vi "UHR-Fleezers Control (fpga) - 10.3 Troy.vi"() -> ()   [LabVIEW 2013]
doc: "UHR-Fleezers Instrument Control Code (fpga)"
uses:
  <vilib>/Platform/TimedLoop/XDataNode/timing_clust.ctl
  <vilib>/Platform/TimedLoop/XDataNode/nitl_modes.ctl
  <vilib>/Platform/TimedLoop/XDataNode/wakeup.ctl
  <vilib>/rvi/eio/common/nirviEmuTemplateMethod_errors.vi
  <vilib>/rvi/Emulation/niFpgaSctlEmulationGetInTimedLoop.vi
  <vilib>/rvi/Emulation/niFpgaEmulationReportErrorSimple.vi
  <vilib>/rvi/Emulation/niFpgaGetClockAttributes.vi
  <vilib>/rvi/Emulation/niFpgaCriticalErrorInLSC.vi
  <vilib>/rvi/Emulation/niFpgaProcessEmulError.vi
  <vilib>/rvi/interface/RandomDataEmulation/nirviRandomDataFPGAFIFO.vi
  <vilib>/rvi/interface/RandomDataEmulation/niFpgaRandomDataHandleErrors.vi
  <vilib>/Platform/TimedLoop/XDataNode/XDataNode.xnode
  <vilib>/eio/EIOMethodNode/EIOMethodNode.xnode
  <vilib>/eio/EIONode/EIONode.xnode
  <vilib>/rvi/DataTransferAndStorage/Container/XNode/niFpgaContainer.xnode
  <vilib>/rvi/interface/RandomDataEmulation/nirviRandomDataFpgaReadWriteTemplate.vi
  <vilib>/addons/control/pid/fpga.llb/XNode/niFpgaPID.xnode
  <vilib>/Platform/TimedLoop/XDataNode/XDNodeRunTimeDep.lvlib
panel:
  out "Trap Pos FB Int-Norm Signal":fxp<+/-,16,1> format="%.16g"
  out "Trap Pos FB Int Signal":fxp<+/-,24,9> format="%.18g"
  in  "Tab Control":T1(tab)
  in  "AI1 X Scale":u16
  in  "Trap Pos FB Monitor T1 or T2":bool
  in  "Trap Pos FB Negate Action":bool
  in  "Trap Pos. FB SP":fxp<+/-,16,1>
  in  "Trap Pos. FB Reset":bool
  in  "Trap Pos to FIFO":bool
  in  "AI1 Sets to FIFO":T2={"Set 1"=TRUE, "Set 2"=TRUE, "Set 3"=FALSE}
  in  "N of AI1 Int Acq Sets":i16=2 min=1 max=3 step=1
  out "AI Late Counter":u16
  in  "ai count":u32=400
  out "AI late?":bool
  in  "+ phase":bool
  in  "Phase count adjustment":i16
  out "Relative phase":i16
  in  "AI to FIFO":bool
  out "BD1 Frequency Out 1":u64
  out "BD1 Frequency Out 2":u64
  in  "Force feedback":bool
  out "AI1 X Set 1":fxp<+/-,16,1>
  in  "Trap Pos. FB Gains":T3={"proportional gain (Kc)"=0.0, "integral gain (Kc*Ts/Ti)"=10.0, "derivative gain (Kc*Td/Ts)"=0.0} {"proportional gain (Kc)" format="%.11g"; "integral gain (Kc*Ts/Ti)" format="%.11g"; "derivative gain (Kc*Td/Ts)" format="%.11g"}
  in  "Trap Pos. FB Range":T4={"output high"=0.999969482421875, "output low"=-1.0}
  in  "Trap Pos. FB Mult Factor":i64=2
  in  "Trap Pos. FB Offset Factor":i64
  out "AI1 X Set 2":fxp<+/-,16,1>
  out "Trap Pos FB Action":i64
  out "Trap Pos FIFO Timeout":u16
  out "Trap AI FIFO Timeout":u16
  in  "Trap FIFO Set Timeout":i32
  in  "Trap Pos FB Int Count":u16=100
  in  "Tab Control 2":T5(tab)
  in  "Swap F1 and F2":bool
  in  "Freq or Amp switch first":bool=TRUE
  in  "Cont. Scan":bool
  in  "Abort scan":bool
  in  "Cycles per step":u64
  in  "Scan BD":bool
  in  "Number of scans":u16
  in  "Scan steps":u64
  in  "Scan freq.  increment":i64
  out "Scanning":bool
  in  "Start scan":bool
  in  "OSK Bd 1":bool
  in  "Reset Bd 1":bool
  in  "RD":bool
  in  "PMODE":bool
  in  "OSK Bd 2":bool
  in  "Reset Bd 2":bool
  in  "Direct RF Box \nCommunication":bool
  in  "Data BD 2":u8 format="%08b"
  in  "Data BD 1":u8 format="%08b"
  in  "Address":u8 format="%02x"
  in  "Update Data":bool
  in  "FPGA Controls\n RF Box":bool
  in  "Number Interlace Cycles":u8=2 min=1 max=3
  in  "Interlace Off Parameters":u8=1 min=1 max=3
  in  "Interlace ON/OFF":bool
  out "DIO Relative phase":i16
  in  "Phase count adjustment (DIO)":i16
  in  "+ phase (DIO)":bool
  out "DIO Late Counter":u16
  out "DIO Late?":bool
  in  "DIO count 1 (ticks)":u32=400
  in  "DIO count 2 (ticks)":u32=400
  in  "DIO count 3 (ticks)":u32=400
  out "AI2 Y Sum Set 2":i16
  out "AI2 Y Sum Set 1":i16
  in  "FB Gains Set 1":T6={"proportional gain (Kc)"=10, "integral gain (Kc*Ts/Ti)"=5, "derivative gain (Kc*Td/Ts)"=0}
  in  "FB Setpoint Set 1":i16 min=0 step=1
  in  "FB Reset Set 1":bool
  in  "FB On/Off Set 1":bool
  in  "FB Reset Set 2":bool
  in  "FB On/Off Set 2":bool
  in  "FB Setpoint Set 2":i16 min=0 step=1
  in  "FB Gains Set 2":T6={"proportional gain (Kc)"=10, "integral gain (Kc*Ts/Ti)"=5, "derivative gain (Kc*Td/Ts)"=0}
  in  "FB output range 2":cluster{"output high":i16, "output low":i16}={"output high"=3000, "output low"=0}
  in  "FB output range 1":cluster{"output high":i16, "output low":i16}={"output high"=3000, "output low"=0}
  out "Scan I":u64
  in  "Amp switch delay":u16=5
  in  "Freq switch delay":u16
  in  "BD 2 Amplitude 1":u16
  in  "BD 1 Amplitude 1":u16
  in  "BD 2 Frequency 1":u64
  in  "BD 1 Frequency 1":u64
  in  "BD 2 Amplitude 2":u16
  in  "BD 1 Amplitude 2":u16
  in  "BD 2 Frequency 2":u64
  in  "BD 1 Frequency 2":u64
  in  "BD 2 Amplitude 3":u16
  in  "BD 1 Amplitude 3":u16
  in  "BD 2 Frequency 3":u64
  in  "BD 1 Frequency 3":u64
  out "Numeric":i32
  out "AO2 2":i16
  out "AO1 2":i16
  in  "1D or 2D Scan?":bool
  in  "Abort scan (MCL)":bool
  in  "MCL Scan Axis":bool
  in  "Cont. Scan (MCL)":bool
  out "Scan I (MCL)":u64
  in  "Number of scans (MCL)":u16
  out "Scanning MCL":bool
  in  "Scan steps (MCL)":u64
  in  "Cycles per step (MCL)":u64
  in  "Scan freq.  increment (MCL)":i16
  in  "Start scan (MCL)":bool
  in  "AO2":i16
  in  "AO1":i16
  out "MCL Late Counter":u16
  out "MCL Late?":bool
  in  "MCL count":u32=800
  out "MCL Relative Phase":i16
  in  "Phase count adjustment (MCL)":i16
  in  "+ phase (MCL)":bool
  in  "APD Gate Operating Mode":u8 max=2 step=1
  in  "Invert APD Gate":bool
  in  "APD Gate OFF Count":u32=100
  in  "APD Gate ON Count":u32=300
  out "APD 1 Gate Late Counter":u16
  out "APD 1 Gate Late?":bool
  out "APD 1 Gate Relative Phase":i16
  in  "Phase count adjustment (APD 1 Gate)":i16
  in  "+ phase (APD 1 Gate)":bool
  out "APD 2 Counts 0":u32
  out "APD 2 Counts 1":u32
  out "APD 1 Counts 0":u32
  out "APD 1 Counts 1":u32
  out "APD1 out state":bool
  in  "APD 2 AO scale factor":i16=1
  in  "APD 1 AO scale factor":i16=1
  in  "APD to FIFO":bool
  in  "APD Acq Rate Count":u32=20000000
  out "APD Acq Late Counter":u16
  out "APD Acq Late?":bool
  out "APD Acq Relative Phase":i16
  in  "Phase Count Adjustment (APD Acq)":i16
  in  "+ phase (APD Acq)":bool
  in  "Phase count adjustment (APD 2 Gate)":i16
  out "APD 2 Gate Late Counter":u16
  out "APD 2 Gate Late?":bool
  out "APD 2 Gate Relative Phase":i16
  in  "+ phase (APD 2 Gate)":bool
  out "APD2 out state":bool
  in  "Green Filter Flipper":bool
  out "Green FB Signals":T7
  in  "Green FB Count":u32=1200
  out "Green Late Counter":u16
  out "Green FB Late?":bool
  out "Green FB Relative Phase":i16
  in  "Phase count adjustment (Green FB)":i16=10
  in  "+ phase (Green FB)":bool
  out "Green FB Sum":i16
  in  "Green int current ON count adj":u32=150
  in  "Current Out":u16=30000
  in  "Green FB On/Off":bool
  in  "Green FB Setpoint":i16=250 min=0 step=1
  in  "Green FB Gains":T6={"proportional gain (Kc)"=10, "integral gain (Kc*Ts/Ti)"=5, "derivative gain (Kc*Td/Ts)"=0}
  in  "Green FB Reset":bool
  in  "Operating Mode 2":u8=2 max=2 step=1
  in  "Invert GI 2":bool
  in  "Green interlace OFF count 2":u32=900
  in  "Green interlace ON count 2":u32=300
  out "GI Late Counter 2":u16
  out "GI Late? 2":bool
  out "GI Relative phase 2":i16
  in  "Phase count adjustment (GI) 2":i16=20
  in  "+ phase (GI) 2":bool
  in  "Green interlace OFF count":u32=100
  out "GI Relative phase":i16
  in  "Phase count adjustment (GI)":i16
  in  "+ phase (GI)":bool
  out "GI Late?":bool
  in  "Green interlace ON count":u32=300
  out "GI Late Counter":u16
  in  "Invert GI":bool
  in  "Operating Mode":u8 max=2 step=1
  in  "Chassis2/Mod4/AO1":u16
  # "Only one of these can be on\nat a time:"
  # "Raster Scan AOD"
  # "1 (X)"
  # "2 (Y)"
  # "IR Intensity Feedback (RF BD 1)"
  # "AO1 (Y)"
  # "2D"
  # "1D"
  # "AO2 (X)"
  # "APD AO for aligning"
  # "Detection Loop"
  # "Green fluorescent laser digital gate interlacing loop"
  # "0 Forced ON\n1 Forced OFF\n2 Interlacing"
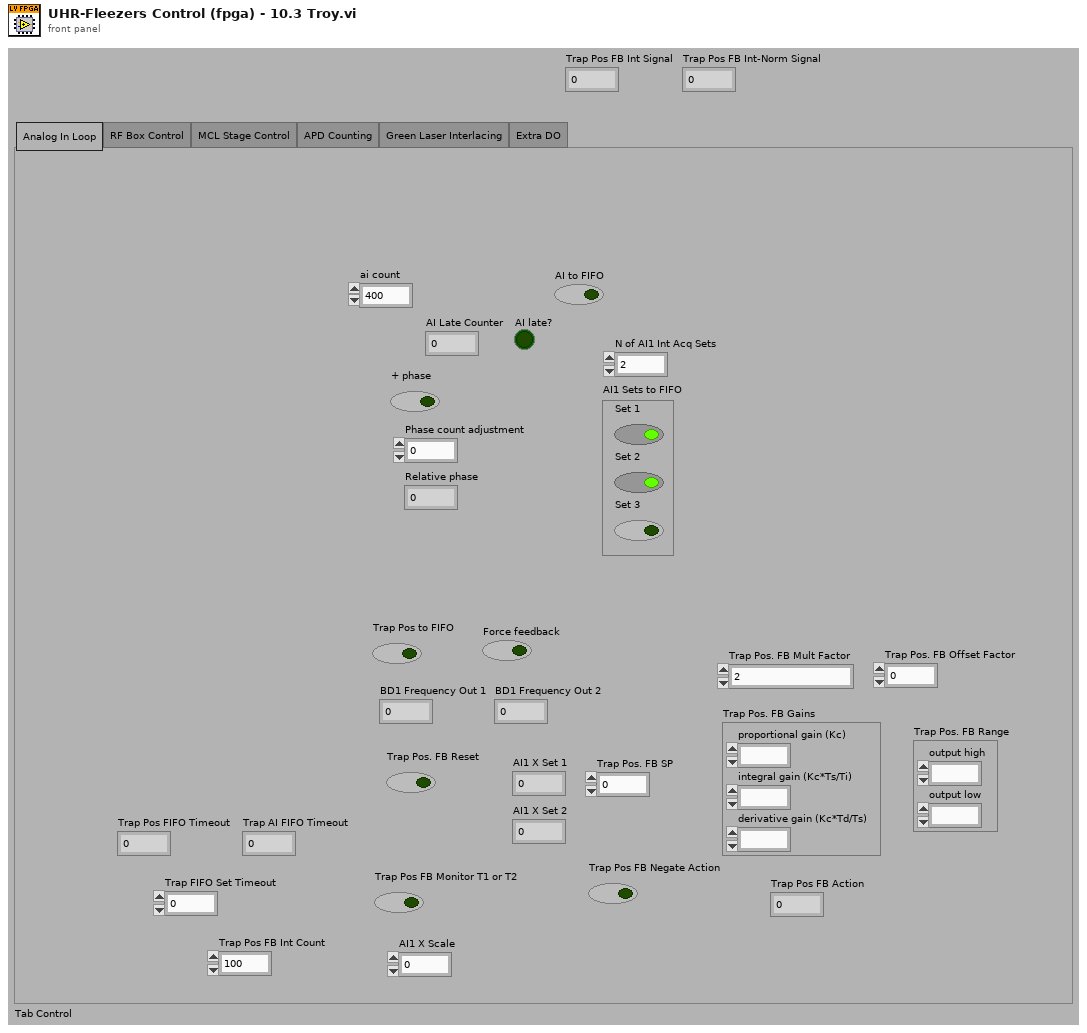
[diagram p1: front panel]
types:
  T1 = enum32{"Analog In Loop", "RF Box Control", "MCL Stage Control", "APD Counting", "Green Laser Interlacing", "Extra DO"}
  T2 = cluster{"Set 1":bool, "Set 2":bool, "Set 3":bool}
  T3 = cluster{"proportional gain (Kc)":fxp<+/-,16,8>, "integral gain (Kc*Ts/Ti)":fxp<+/-,16,8>, "derivative gain (Kc*Td/Ts)":fxp<+/-,16,8>}
  T4 = cluster{"output high":fxp<+/-,16,1>, "output low":fxp<+/-,16,1>}
  T5 = enum32{"Controls", "Interlacing Frequency and Amplitude Values"}
  T6 = cluster{"proportional gain (Kc)":i16, "integral gain (Kc*Ts/Ti)":i16, "derivative gain (Kc*Td/Ts)":i16}
  T7 = cluster{"Green FB Ch 0":i16, "Green FB Ch 1":i16, "Green FB Ch 2":i16}
  T8 = typedef "XDNodeRunTimeDep.lvlib/timing_clust.ctl" = cluster{"Expected End [f-1]":u64, "Actual End [f-1]":u64, "Finished Late? [f-1]":bool, "Expected End [i-1]":u64, "Actual End [i-1]":u64, "Finished Late? [i-1]":bool, "Expected Start [i]":u64, "Actual Start [i]":u64, "Expected Start [f]":u64, "Actual Start [f]":u64, "Source Name":string, "Structure Name":string, "Period":i64, "Deadline":i64, "Offset":i64, "Start":i64, "Priority":i32, "Timeout":i32, "Mode":T9, "Wakeup Reason":T10, "Error":errorcluster, "Source Type":string, "Secondary Source Type":string, "Global End Time":u64, "Global Start Time":u64, "Frame Duration":u64, "Iteration Duration":u64, "Assigned CPU":i32, "I/O Scan Engine Mode":u32}
  T9 = typedef "XDNodeRunTimeDep.lvlib/nitl_modes.ctl" = enum32{"No Change", "Process missed periods, maintain original phase", "Discard missed periods, maintain original phase", "Process missed periods, ignore original phase", "Discard missed periods, ignore original phase"}
  T10 = typedef "XDNodeRunTimeDep.lvlib/wakeup.ctl" = enum32{"Normal", "Aborted", "Asynchronous wakeup", "Timing source error", "Timed loop error", "Timeout"}
  T11 = cluster{"Chassis2/Mod2/AI0":i16, "Chassis2/Mod2/AI1":i16, "Chassis2/Mod2/AI2":i16}
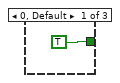
[diagram p2: hidden frame]
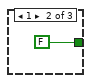
[diagram p3: hidden frame]
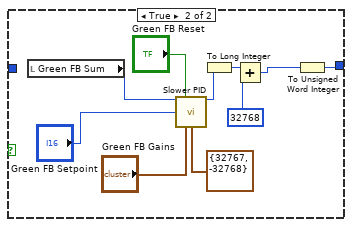
[diagram p4: hidden frame]
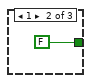
[diagram p5: hidden frame]
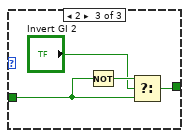
[diagram p6: hidden frame]
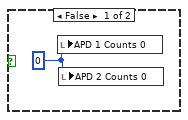
[diagram p7: hidden frame]
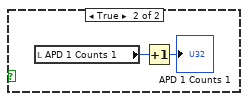
[diagram p9: hidden frame]
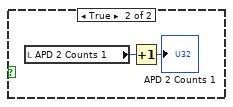
[diagram p10: hidden frame]
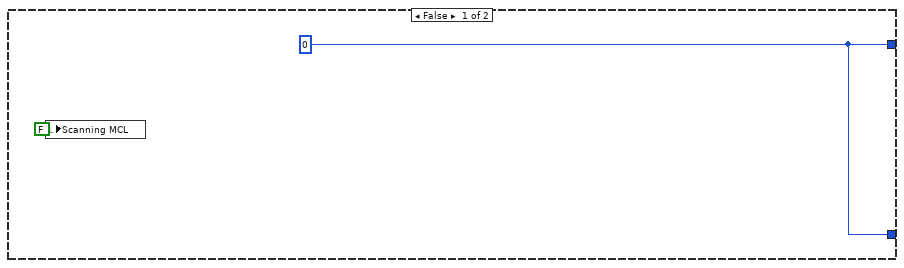
[diagram p11: hidden frame]
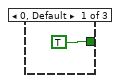
[diagram p12: hidden frame]
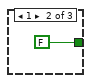
[diagram p13: hidden frame]
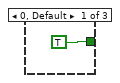
[diagram p14: hidden frame]
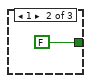
[diagram p15: hidden frame]
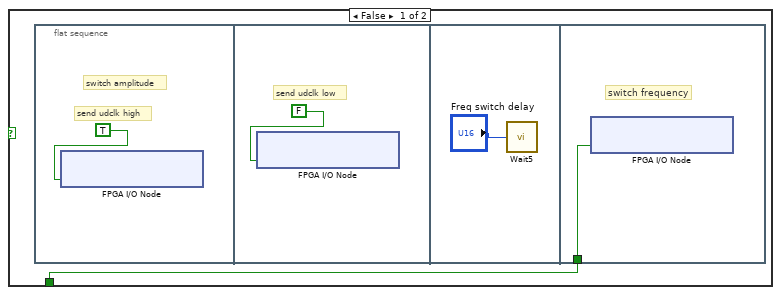
[diagram p18: hidden frame]
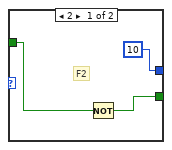
[diagram p20: hidden frame]
diagram:
  w3 = FALSE
  # "timing array current index"
  # "timing array"
  # "timing counter (phase adjusted here)"
  # "late counter"
  n1 = flat-sequence "FPGA initialization to do before running any of the loops" {
    tunnel: [u32 0 ("DIO count 3 (ticks)")] -> w2
    tunnel: [w10] -> _
    frame #0 {
      # "Start up expansion chassis early\nto avoid delays later"
      # "This pin controls udclk on the RF boards.\nWhen initially configuring the boards, this pin needs to be\nconfigured as a high impedance input.  Later it will be switched\nto an output."
      # "Initial setting of DIO data and \naddress to low (before reset).  \nThis needs to happen before the other\ncontrol method loops execute."
      n2 = xnode "FPGA I/O Node"("Connector1/DIO0"=FALSE, "Connector1/DIO1"=FALSE, "Connector1/DIO2"=FALSE, "Connector1/DIO3"=FALSE, "Connector1/DIO4"=FALSE, "Connector1/DIO5"=FALSE, "Connector1/DIO6"=FALSE, "Connector1/DIO7"=FALSE, "Connector1/DIO8"=FALSE, "Connector1/DIO9"=FALSE, "Connector1/DIO10"=FALSE, "Connector1/DIO11"=FALSE, "Connector1/DIO12"=FALSE, "Connector1/DIO13"=FALSE, "Connector1/DIO15"=FALSE, "Connector1/DIO20"=FALSE, "Connector1/DIO21"=FALSE, "Connector1/DIO22"=FALSE, "Connector1/DIO23"=FALSE, "Connector1/DIO24"=FALSE, "Connector1/DIO25"=FALSE, "Connector1/DIO26"=FALSE, "Connector1/DIO27"=FALSE, "Connector1/DIO14"=FALSE) -> ()  [unwired: 24 in, 24 out]
      n3 = xnode "FPGA I/O Method Node"("Enable"=FALSE) -> ()  [unwired: 1 in, 1 out]
      n4 = xnode "FPGA I/O Node"("Chassis2/Mod1/AO0"=u16 0 ("Chassis2/Mod4/AO0")) -> ("Chassis2/Mod2/AI0"=w10:i16)  [unwired: 2 in, 2 out]
    }
  }
  n5 = local read "AO1"() -> (w7:i16)
  n6 = local read "AO2"() -> (w6:i16)
  n7 = node-c288() -> (w5:T8)  [unwired: 1 in]
  n8 = while "APD 1 Counter" {
    tunnel: w2 -> [_]
    stop <- FALSE stop-if-true
    n9 = flat-sequence {
      frame #0 {
        n10 = xnode "FPGA I/O Method Node"("FPGA I/O In"=refnum<k21> "Connector0/DIO0" ("APD 1 DO"), "Timeout"=-1) -> ()  [unwired: 2 out]
      }
      frame #1 {
        n11 = local read "APD1 out state"() -> (w41:bool)
        n12 = case shown="False" w41 {
          frame False {
            n13 = local read "APD 1 Counts 0"() -> (w43:u32)
            n14 = Increment(x=w43) -> (x+1=→"APD 1 Counts 0":u32)
          }
          frame True {
            n15 = local read "APD 1 Counts 1"() -> (w45:u32)
            n16 = Increment(x=w45) -> (x+1=→"APD 1 Counts 1":u32)
          }
        }
      }
    }
  }
  n17 = while "APD 2 Counter" {
    tunnel: w2 -> [_]
    stop <- FALSE stop-if-true
    n18 = flat-sequence {
      frame #0 {
        n19 = xnode "FPGA I/O Method Node"("FPGA I/O In"=refnum<k21> "Connector0/DIO1" ("APD 2 DO"), "Timeout"=-1) -> ()  [unwired: 2 out]
      }
      frame #1 {
        n20 = local read "APD2 out state"() -> (w49:bool)
        n21 = case shown="False" w49 {
          frame False {
            n22 = local read "APD 2 Counts 0"() -> (w51:u32)
            n23 = Increment(x=w51) -> (x+1=→"APD 2 Counts 0":u32)
          }
          frame True {
            n24 = local read "APD 2 Counts 1"() -> (w53:u32)
            n25 = Increment(x=w53) -> (x+1=→"APD 2 Counts 1":u32)
          }
        }
      }
    }
  }
  n26 = timed-loop "RF box board DIO control: control bits" {
    timing: w5 -> [_]
    timing-out: [_] -> w4
    tunnel: [w54] -> _
    tunnel: w2 -> [w54]
    stop <- FALSE stop-if-true
    n27 = xnode "FPGA I/O Node"("Connector1/DIO16"="RD", "Connector1/DIO17"="PMODE", "Connector1/DIO18"="OSK Bd 1", "Connector1/DIO19"="Reset Bd 1", "Connector1/DIO28"="OSK Bd 2", "Connector1/DIO29"="Reset Bd 2") -> ()  [unwired: 6 in, 6 out]
  }
  n28 = while "Control Additional IO (Green laser flip mount)" {
    stop <- FALSE stop-if-true
    n29 = xnode "FPGA I/O Node"("Connector0/DIO3"="Green Filter Flipper", "Chassis2/Mod1/AO1"="Chassis2/Mod4/AO1") -> ()  [unwired: 2 in, 2 out]
    n30 = call "Loop Timer2"("Count(Ticks)"=u32 40000 ("Extra DO Counts")) -> ()  [unwired: 1 out]
  }
  n31 = while "RF box board direct communication loop" {
    tunnel: w2 -> [_]
    stop <- FALSE stop-if-true
    n32 = case "Whether to use direct communication method (only use one method at a time)" shown="True" "Direct RF Box \nCommunication" {
      frame False {
      }
      frame True {
        n33 = case shown="True" "Update Data" {
          frame False {
          }
          frame True {
            n34 = flat-sequence {
              frame #0 {
                n35 = First Call?() -> (First Call?: T/F=w71:bool)
                n36 = case shown="True" w71 {
                  frame False {
                  }
                  frame True {
                    # "If first time data updated, be sure to set WR high\nbefore setting data and address bits."
                    n37 = flat-sequence {
                      frame #0 {
                        n38 = xnode "FPGA I/O Node"("Connector1/DIO15"=TRUE) -> ()  [unwired: 1 in, 1 out]
                      }
                      frame #1 {
                        n39 = call "Wait"("Count(Ticks)"=u8 40 ("DO Delay 3 (Ticks)")) -> ()  [unwired: 1 out]
                      }
                    }
                  }
                }
              }
              frame #1 {
                n40 = Number To Boolean Array(number="Address") -> (Boolean array=w120:bool[])
                n41 = Number To Boolean Array(number="Data BD 1") -> (Boolean array=w121:bool[])
                n42 = Number To Boolean Array(number="Data BD 2") -> (Boolean array=w90:bool[])
                n43 = Index Array(array=w121, index=7) -> (element=w105:bool)
                n44 = Index Array(array=w121, index=6) -> (element=w104:bool)
                n45 = Index Array(array=w121, index=5) -> (element=w103:bool)
                n46 = Index Array(array=w121, index=4) -> (element=w102:bool)
                n47 = Index Array(array=w121, index=3) -> (element=w101:bool)
                n48 = Index Array(array=w121, index=2) -> (element=w100:bool)
                n49 = Index Array(array=w121, index=1) -> (element=w99:bool)
                n50 = Index Array(array=w121, index=0) -> (element=w98:bool)
                n51 = Index Array(array=w120, index=5) -> (element=w97:bool)
                n52 = Index Array(array=w120, index=4) -> (element=w96:bool)
                n53 = Index Array(array=w120, index=3) -> (element=w95:bool)
                n54 = Index Array(array=w120, index=2) -> (element=w94:bool)
                n55 = Index Array(array=w120, index=1) -> (element=w93:bool)
                n56 = Index Array(array=w120, index=0) -> (element=w92:bool)
                n57 = Index Array(array=w90, index=7) -> (element=w81:bool)
                n58 = Index Array(array=w90, index=6) -> (element=w80:bool)
                n59 = Index Array(array=w90, index=5) -> (element=w79:bool)
                n60 = Index Array(array=w90, index=4) -> (element=w78:bool)
                n61 = Index Array(array=w90, index=3) -> (element=w77:bool)
                n62 = Index Array(array=w90, index=2) -> (element=w76:bool)
                n63 = Index Array(array=w90, index=1) -> (element=w75:bool)
                n64 = Index Array(array=w90, index=0) -> (element=w74:bool)
                n65 = xnode "FPGA I/O Node"("Connector1/DIO0"=w105, "Connector1/DIO1"=w104, "Connector1/DIO2"=w103, "Connector1/DIO3"=w102, "Connector1/DIO4"=w101, "Connector1/DIO5"=w100, "Connector1/DIO6"=w99, "Connector1/DIO7"=w98, "Connector1/DIO8"=w97, "Connector1/DIO9"=w96, "Connector1/DIO10"=w95, "Connector1/DIO11"=w94, "Connector1/DIO12"=w93, "Connector1/DIO13"=w92, "Connector1/DIO20"=w81, "Connector1/DIO21"=w80, "Connector1/DIO22"=w79, "Connector1/DIO23"=w78, "Connector1/DIO24"=w77, "Connector1/DIO25"=w76, "Connector1/DIO26"=w75, "Connector1/DIO27"=w74) -> ()  [unwired: 22 in, 22 out]
              }
              frame #2 {
                # "wait and then apply write signal"
                n66 = call "Wait2"("Count(Ticks)"=u8 40 ("DO Delay 1 (Ticks)")) -> ()  [unwired: 1 out]
              }
              frame #3 {
                # "sending bit low writes data to board buffer"
                n67 = xnode "FPGA I/O Node"("Connector1/DIO15"=FALSE) -> ()  [unwired: 1 in, 1 out]
              }
              frame #4 {
                # "wait then return write signal"
                n68 = call "Wait3"("Count(Ticks)"=u8 40 ("DO Delay 2 (Ticks)")) -> ()  [unwired: 1 out]
              }
              frame #5 {
                # "sending bit high makes ready to\nwrite more data"
                n69 = xnode "FPGA I/O Node"("Connector1/DIO15"=TRUE) -> ()  [unwired: 1 in, 1 out]
              }
            }
          }
        }
      }
    }
  }
  n70 = while "APD 2 Gating" {
    shift-right: [w131] -> _
    shift-left: w2 -> [w136]
    shift-right: [w130] -> _
    shift-left: w3 -> [w128]
    stop <- FALSE stop-if-true
    n71 = flat-sequence {
      tunnel: w136 -> [w139]
      tunnel: [w140] -> w134
      tunnel: [w139] -> w132
      tunnel: [w138] -> w129
      tunnel: w128 -> [w138]
      tunnel: [w143] -> w135
      tunnel: w134 -> [w143]
      tunnel: [w142] -> w133
      tunnel: w132 -> [w142]
      tunnel: w129 -> [w141]
      tunnel: [w161] -> w131
      tunnel: w135 -> [w172]
      tunnel: w133 -> [w170]
      tunnel: [w165] -> w130
      frame #0 {
        n72 = call "Loop Timer8"("Count(Ticks)"=w139) -> ("Tick Count(Ticks)"=w140:u32)
      }
      frame #1 {
        # "(need 4 channels/APD)"
        n73 = xnode "FPGA I/O Node"("Connector1/DIO26"=w141, "Connector1/DIO27"=w141, "Connector1/DIO22"=w141, "Connector1/DIO32"=w141, "Connector1/DIO34"=w141, "Connector1/DIO33"=w141, "Connector1/DIO35"=w141) -> ()  [unwired: 7 in, 7 out]
      }
      frame #2 {
        n74 = local read "APD Gate ON Count"() -> (w154:u32)
        n75 = local read "APD Gate OFF Count"() -> (w153:u32)
        n76 = feedback #1(TRUE) -> (w167:bool)
        n77 = feedback-in #2(w172) -> ()
        n78 = feedback #2(w172) -> (w155:u32)
        n79 = Not(x=w167) -> (.not. x?=w164:bool)
        n80 = feedback-in #1(w164) -> ()
        n81 = Subtract(x=w172, y=w155) -> (x-y=w171:u32)
        n82 = Select(t=w154, s=w164, f=w153) -> (s? t:f=w169:u32)
        n83 = Subtract(x=w171, y=w170) -> (x-y=w146:u32)
        n84 = Subtract(x=w169, y=w146) -> (x-y=w160:u32)
        n85 = Number To Boolean Array(number=w146) -> (Boolean array=w145:bool[])
        n86 = Or Array Elements(Boolean array=w145) -> (logical OR=w144:bool)
        "APD 2 Gate Late?" <- w144
        n87 = Boolean To (0,1)(Boolean="+ phase (APD 2 Gate)") -> (0, 1=w158:i16)
        n88 = Multiply(x=w158, y="Phase count adjustment (APD 2 Gate)") -> (x*y=w156:i16)
        n89 = Boolean To (0,1)(Boolean=w144) -> (0, 1=w151:i16)
        n90 = Add(x=w160, y=w156) -> (x+y=w161:u32)
        n91 = To Unsigned Word Integer(number=w151) -> (unsigned 16bit integer=w148:u16)
        n92 = feedback #3(i16 0) -> (w163:i16)
        n93 = Subtract(x=w163, y=w156) -> (x-y=w162:i16)
        "APD 2 Gate Relative Phase" <- w162
        n94 = feedback-in #3(w162) -> ()
        n95 = feedback #4(u16 0) -> (w149:u16)
        n96 = Add(x=w148, y=w149) -> (x+y=w147:u16)
        "APD 2 Gate Late Counter" <- w147
        n97 = feedback-in #4(w147) -> ()
        n98 = local read "APD Gate Operating Mode"() -> (w152:u8)
        n99 = case shown="2" w152 {
          tunnel: [TRUE FALSE w178] -> w165
          tunnel: w167 -> [_ _ w176]
          frame 0, Default {
          }
          frame 1 {
          }
          frame 2 {
            n100 = local read "Invert APD Gate"() -> (w175:bool)
            n101 = Not(x=w176) -> (.not. x?=w177:bool)
            n102 = Select(t=w177, s=w175, f=w176) -> (s? t:f=w178:bool)
          }
        }
      }
    }
  }
  n103 = while "APD 1 Gating" {
    shift-right: [w182] -> _
    shift-left: w2 -> [w187]
    shift-right: [w181] -> _
    shift-left: w3 -> [w179]
    stop <- FALSE stop-if-true
    n104 = flat-sequence {
      tunnel: w187 -> [w190]
      tunnel: [w191] -> w185
      tunnel: [w190] -> w183
      tunnel: [w189] -> w180
      tunnel: w179 -> [w189]
      tunnel: [w194] -> w186
      tunnel: w185 -> [w194]
      tunnel: [w193] -> w184
      tunnel: w183 -> [w193]
      tunnel: w180 -> [w192]
      tunnel: [w208] -> w182
      tunnel: w186 -> [w223]
      tunnel: w184 -> [w220]
      tunnel: [w212] -> w181
      frame #0 {
        n105 = call "Loop Timer7"("Count(Ticks)"=w190) -> ("Tick Count(Ticks)"=w191:u32)
      }
      frame #1 {
        # "(need 4 channels/APD)"
        n106 = xnode "FPGA I/O Node"("Connector0/DIO8"=w192, "Connector0/DIO9"=w192, "Connector0/DIO10"=w192, "Connector0/DIO11"=w192, "Connector0/DIO4"=w192, "Connector0/DIO5"=w192, "Connector0/DIO6"=w192, "Connector0/DIO7"=w192) -> ()  [unwired: 8 in, 8 out]
      }
      frame #2 {
        n107 = feedback #5(TRUE) -> (w215:bool)
        n108 = feedback-in #6(w223) -> ()
        n109 = feedback #6(w223) -> (w222:u32)
        n110 = Not(x=w215) -> (.not. x?=w211:bool)
        n111 = feedback-in #5(w211) -> ()
        n112 = Subtract(x=w223, y=w222) -> (x-y=w221:u32)
        n113 = Select(t="APD Gate ON Count", s=w211, f="APD Gate OFF Count") -> (s? t:f=w217:u32)
        n114 = Subtract(x=w221, y=w220) -> (x-y=w196:u32)
        n115 = Subtract(x=w217, y=w196) -> (x-y=w207:u32)
        n116 = Number To Boolean Array(number=w196) -> (Boolean array=w197:bool[])
        n117 = Or Array Elements(Boolean array=w197) -> (logical OR=w195:bool)
        "APD 1 Gate Late?" <- w195
        n118 = Boolean To (0,1)(Boolean="+ phase (APD 1 Gate)") -> (0, 1=w205:i16)
        n119 = Boolean To (0,1)(Boolean=w195) -> (0, 1=w202:i16)
        n120 = Multiply(x=w205, y="Phase count adjustment (APD 1 Gate)") -> (x*y=w203:i16)
        n121 = To Unsigned Word Integer(number=w202) -> (unsigned 16bit integer=w199:u16)
        n122 = Add(x=w207, y=w203) -> (x+y=w208:u32)
        n123 = feedback #7(i16 0) -> (w210:i16)
        n124 = Subtract(x=w210, y=w203) -> (x-y=w209:i16)
        "APD 1 Gate Relative Phase" <- w209
        n125 = feedback-in #7(w209) -> ()
        n126 = feedback #8(u16 0) -> (w200:u16)
        n127 = Add(x=w199, y=w200) -> (x+y=w198:u16)
        "APD 1 Gate Late Counter" <- w198
        n128 = feedback-in #8(w198) -> ()
        n129 = case shown="2" "APD Gate Operating Mode" {
          tunnel: [TRUE FALSE w229] -> w212
          tunnel: w215 -> [_ _ w226]
          frame 0, Default {
          }
          frame 1 {
          }
          frame 2 {
            n130 = Not(x=w226) -> (.not. x?=w228:bool)
            n131 = Select(t=w228, s="Invert APD Gate", f=w226) -> (s? t:f=w229:bool)
          }
        }
      }
    }
  }
  n132 = while "DAQ AI set 1" {
    shift-right: [w230] -> _
    shift-left: w2 -> [w235]
    stop <- FALSE stop-if-true
    n133 = flat-sequence {
      tunnel: w235 -> [w245]
      tunnel: [w246] -> w233
      tunnel: [w245] -> w232
      tunnel: [w256] -> w243
      tunnel: [w255] -> w242
      tunnel: [w254] -> w241
      tunnel: [w253] -> w240
      tunnel: [w252] -> w239
      tunnel: [w251] -> w238
      tunnel: [w250] -> w237
      tunnel: [w249] -> w236
      tunnel: [w248] -> w234
      tunnel: w233 -> [w248]
      tunnel: w232 -> [w247]
      tunnel: [w247] -> w231
      tunnel: [w285] -> w230
      tunnel: w243 -> [w313]
      tunnel: w242 -> [w277]
      tunnel: w241 -> [w278]
      tunnel: w240 -> [w312]
      tunnel: w239 -> [w301]
      tunnel: w238 -> [w300]
      tunnel: w237 -> [w299]
      tunnel: w236 -> [w298]
      tunnel: w234 -> [w295]
      tunnel: w231 -> [w292]
      frame #0 {
        n134 = call "Loop Timer3"("Count(Ticks)"=w245) -> ("Tick Count(Ticks)"=w246:u32)
      }
      frame #1 {
        # "detection \nlaser qpd"
        # "sum"
        # "x"
        # "y"
        # "1064 int\nfeedback qpd"
        # "sum"
        # "x"
        # "traps\nqpd"
        # "sum"
        # "y"
        # "x"
        n135 = xnode "FPGA I/O Node"("Connector1/DIO31"=TRUE ("Connector1/DIO33")) -> ("Connector0/AI0"=w256:i16, "Connector0/AI1"=w255:i16, "Connector0/AI2"=w254:i16, "Connector0/AI3"=w253:i16, "Connector0/AI4"=w252:i16, "Connector0/AI5"=w251:i16, "Connector0/AI6"=w250:i16, "Connector0/AI7"=w249:i16)  [unwired: 9 in, 9 out]
      }
      frame #2 {
        w281 = FALSE ("AI to FIFO")
        # "only write specified sets (1 and 2 usually) to FIFO \nif AI to FIFO is true"
        # "Adjust phase after data acquired if button pressed"
        n136 = feedback #9(i16 1) -> (w305:i16)
        n137 = Increment(x=w305) -> (x+1=w311:i16)
        n138 = Scale By Power Of 2(n="AI1 X Scale", x=w277) -> (x*2^n=w275:i16)
        n139 = Greater?(x=w311, y="N of AI1 Int Acq Sets") -> (0:w308:bool)
        n140 = Divide(x=w275, y=w278) -> (x/y=w274:fxp<+/-,16,1>)
        n141 = Select(t=i16 1, s=w308, f=w311) -> (s? t:f=w310:i16)
        n142 = feedback-in #9(w310) -> ()
        n143 = feedback #10(w281) -> (w279:bool)
        n144 = feedback #11(w281) -> (w297:bool)
        n145 = case shown="1, Default" w305 {
          tunnel: w278 -> [w335 w343 _]
          tunnel: "AI1 Sets to FIFO" -> [w339 w347 w353]
          tunnel: [w338 w346 w352] -> w302
          tunnel: ["AI to FIFO" w345 w351] -> w296
          tunnel: w297 -> [_ w345 w351]
          tunnel: ["Trap Pos to FIFO" w344 w350] -> w280
          tunnel: w279 -> [_ w344 w350]
          tunnel: w274 -> [w334 w342 _]
          tunnel: [w333 w340 FALSE] -> w261
          tunnel: [w332 w341 u64 0 ("BD1 Frequency Out 2")] -> w260
          frame 1, Default {
            n146 = Unbundle By Name(w339) -> ("Set 1"=w338:bool)
            n147 = local read "BD1 Frequency Out 1"() -> (w332:u64)
            n148 = Compound Arithmetic op=AND("Trap Pos to FIFO", w338, "AI to FIFO") -> (w333:bool)
            "AI2 Y Sum Set 1" <- w335
            "AI1 X Set 1" <- w334
          }
          frame 2 {
            n149 = Unbundle By Name(w347) -> ("Set 2"=w346:bool)
            n150 = local read "BD1 Frequency Out 2"() -> (w341:u64)
            n151 = Compound Arithmetic op=AND(w344, w346, w345) -> (w340:bool)
            "AI2 Y Sum Set 2" <- w343
            "AI1 X Set 2" <- w342
          }
          frame 3 {
            n152 = Unbundle By Name(w353) -> ("Set 3"=w352:bool)
          }
        }
        n153 = And(x=w302, y=w296) -> (x .and. y?=w304:bool)
        n154 = feedback-in #10(w280) -> ()
        n155 = case shown="True" w304 {
          tunnel: w313 -> [_ w367]
          tunnel: w277 -> [_ w366]
          tunnel: w278 -> [_ w365]
          tunnel: w312 -> [_ w364]
          tunnel: w301 -> [_ w363]
          tunnel: w300 -> [_ w362]
          tunnel: w299 -> [_ w361]
          tunnel: w298 -> [_ w360]
          tunnel: 0 ("DMA buffer timeout") -> [_ w369]
          frame False {
          }
          frame True {
            n156 = Build Array(w367, w366, w365, w364, w363, w362, w361, w360) -> (w368:i16[])
            n157 = for {
              tunnel: w368 -> [w371] mode=indexing
              tunnel: w369 -> [w372]
              tunnel: [w370] -> w358 mode=indexing
              n158 = xnode ("FIFO Write")("Element"=w371, "Timeout"=w372) -> ("Timed Out?"=w370:bool)  [unwired: 1 in, 1 out]
            }
            n159 = Or Array Elements(Boolean array=w358) -> (logical OR=w355:bool)
            n160 = Boolean To (0,1)(Boolean=w355) -> (0, 1=w357:i16)
            n161 = feedback #12(u16 0) -> (w356:u16)
            n162 = Add(x=w357, y=w356) -> (x+y=w354:u16)
            "Trap AI FIFO Timeout" <- w354
            n163 = feedback-in #12(w354) -> ()
          }
        }
        n164 = feedback-in #11(w296) -> ()
        n165 = case shown="True" w261 {
          tunnel: w260 -> [_ w319]
          tunnel: [u8 0 w316] -> w259
          frame False {
          }
          frame True {
            n166 = Split Number(x=w319) -> (hi(x)=w320:u32, lo(x)=w321:u32)
            n167 = Split Number(x=w320) -> (lo(x)=w322:u16)  [unwired: 1 out]
            n168 = Split Number(x=w321) -> (hi(x)=w323:u16, lo(x)=w324:u16)
            n169 = Build Array "BD 1 nu Stack"(w322, w323, w324) -> (w318:u16[])
            n170 = for {
              tunnel: w318 -> [w331] mode=indexing
              shift-right: [w327] -> w316
              shift-left: u8 0 -> [w328]
              n171 = xnode ("FIFO Method Node")("Element"=w331, "Timeout"="Trap FIFO Set Timeout") -> ("Timed Out?"=w330:bool)  [unwired: 1 in, 1 out]
              n172 = Boolean To (0,1)(Boolean=w330) -> (0, 1=w329:i16)
              n173 = To Unsigned Byte Integer(number=w329) -> (unsigned 8bit integer=w326:u8)
              n174 = Add(x=w326, y=w328) -> (x+y=w327:u8)
            }
          }
        }
        n175 = To Unsigned Word Integer(number=w259) -> (unsigned 16bit integer=w258:u16)
        n176 = feedback #13(u16 0) -> (w272:u16)
        n177 = Add(x=w258, y=w272) -> (x+y=w271:u16)
        "Trap Pos FIFO Timeout" <- w271
        n178 = feedback-in #13(w271) -> ()
        n179 = feedback-in #14(w295) -> ()
        n180 = feedback #14(w295) -> (w294:u32)
        n181 = Subtract(x=w295, y=w294) -> (x-y=w293:u32)
        n182 = xnode "I/O Node"("Connector1/DIO31"=FALSE ("Connector1/DIO34")) -> ()  [unwired: 1 in, 1 out]
        n183 = Subtract(x=w293, y=w292) -> (x-y=w263:u32)
        n184 = Boolean To (0,1)(Boolean="+ phase") -> (0, 1=w288:i16)
        n185 = Multiply(x=w288, y="Phase count adjustment") -> (x*y=w282:i16)
        n186 = Subtract(x="ai count", y=w263) -> (x-y=w286:u32)
        n187 = Number To Boolean Array(number=w263) -> (Boolean array=w264:bool[])
        n188 = feedback #15(i16 0) -> (w284:i16)
        n189 = Add(x=w286, y=w282) -> (x+y=w285:u32)
        n190 = Subtract(x=w284, y=w282) -> (x-y=w283:i16)
        "Relative phase" <- w283
        n191 = feedback-in #15(w283) -> ()
        n192 = Or Array Elements(Boolean array=w264) -> (logical OR=w262:bool)
        "AI late?" <- w262
        n193 = Boolean To (0,1)(Boolean=w262) -> (0, 1=w269:i16)
        n194 = To Unsigned Word Integer(number=w269) -> (unsigned 16bit integer=w266:u16)
        n195 = feedback #16(u16 0) -> (w267:u16)
        n196 = Add(x=w266, y=w267) -> (x+y=w265:u16)
        "AI Late Counter" <- w265
        n197 = feedback-in #16(w265) -> ()
      }
    }
  }
  n198 = while "MCL stage control" {
    shift-right: [w388] -> _
    shift-left: w2 -> [w391]
    shift-right: [w381] -> _
    shift-left: w7 -> [w378]
    shift-right: [w380] -> _
    shift-left: w6 -> [w376]
    i -> [w375]
    stop <- FALSE stop-if-true
    n199 = flat-sequence {
      tunnel: w391 -> [w395]
      tunnel: [w396] -> w387
      tunnel: [w395] -> w385
      tunnel: [w394] -> w379
      tunnel: w378 -> [w394]
      tunnel: [w393] -> w377
      tunnel: w376 -> [w393]
      tunnel: w387 -> [w400]
      tunnel: [w400] -> w386
      tunnel: w385 -> [w399]
      tunnel: [w399] -> w384
      tunnel: w379 -> [w398]
      tunnel: w377 -> [w397]
      tunnel: [w398] -> w374
      tunnel: [w397] -> w373
      tunnel: w386 -> [w410]
      tunnel: w384 -> [w409]
      tunnel: [w410] -> w390
      tunnel: [w409] -> w389
      tunnel: [w408] -> w383
      tunnel: [w407] -> w382
      tunnel: w374 -> [w402]
      tunnel: w373 -> [w401]
      tunnel: [w482] -> w388
      tunnel: w390 -> [w489]
      tunnel: w389 -> [w486]
      tunnel: w383 -> [w484]
      tunnel: w382 -> [w483]
      tunnel: [w484] -> w381
      tunnel: [w483] -> w380
      frame #0 {
        n200 = call "Loop Timer5"("Count(Ticks)"=w395) -> ("Tick Count(Ticks)"=w396:u32)
      }
      frame #1 {
        n201 = xnode "FPGA I/O Node"("Connector0/AO1"=w398, "Connector0/AO2"=w397) -> ()  [unwired: 2 in, 2 out]
      }
      frame #2 {
        n202 = local read "Scanning MCL"() -> (w422:bool)
        n203 = Or(x=w422, y="Start scan (MCL)") -> (x .or. y?=w417:bool)
        n204 = Not(x="Abort scan (MCL)") -> (.not. x?=w415:bool)
        n205 = And(x=w415, y=w417) -> (x .and. y?=w414:bool)
        n206 = case "Raster scan" shown="True" w414 {
          tunnel: [w423 w466] -> w419
          tunnel: "Start scan (MCL)" -> [_ w451]
          tunnel: [w423 w427] -> w403
          frame False {
            w423 = i16 0
            n207 = local write "Scanning MCL"(FALSE ("scanning")) -> ()
          }
          frame True {
            w437 = i16 0
            w436 = u64 0
            # "scan incr."
            # "freq. incr. mult."
            # "count steps"
            # "count number of cycles"
            n208 = feedback #17(w436) -> (w463:u64)
            n209 = Select(t=w436, s=w451, f=w463) -> (s? t:f=w465:u64)
            n210 = Increment(x=w465) -> (x+1=w462:u64)
            n211 = Greater?(x="Cycles per step (MCL)", y=w462) -> (0:w446:bool)
            n212 = Select(t=w462, s=w446, f=w436) -> (s? t:f=w461:u64)
            n213 = feedback-in #17(w461) -> ()
            n214 = feedback #18(w436) -> (w460:u64)
            n215 = Select(t=w436, s=w451, f=w460) -> (s? t:f=w455:u64)
            n216 = Increment(x=w455) -> (x+1=w459:u64)
            n217 = Add(x="Scan steps (MCL)", y="Scan steps (MCL)") -> (x+y=w458:u64)
            n218 = Select(t=w455, s=w446, f=w459) -> (s? t:f=w441:u64)
            n219 = Greater?(x=w458, y=w441) -> (0:w440:bool)
            n220 = Select(t=w441, s=w440, f=w436) -> (s? t:f=w456:u64)
            n221 = feedback-in #18(w456) -> ()
            n222 = Equal?(x="Scan steps (MCL)", y=w441) -> (x = y?=w445:bool)
            n223 = Greater?(x="Scan steps (MCL)", y=w455) -> (0:w454:bool)
            n224 = feedback #19(w437) -> (w457:i16)
            n225 = Select(t=w437, s=w451, f=w457) -> (s? t:f=w443:i16)
            n226 = Increment(x=w443) -> (x+1=w453:i16)
            n227 = Decrement(x=w443) -> (x-1=w452:i16)
            n228 = Select(t=w453, s=w454, f=w452) -> (s? t:f=w444:i16)
            n229 = Select(t=w443, s=w445, f=w444) -> (s? t:f=w442:i16)
            n230 = Select(t=w443, s=w446, f=w442) -> (s? t:f=w438:i16)
            n231 = Select(t=w438, s=w440, f=w437) -> (s? t:f=w439:i16)
            n232 = feedback-in #19(w439) -> ()
            n233 = feedback #20(w436) -> (w450:u64)
            n234 = Select(t=w436, s=w451, f=w450) -> (s? t:f=w425:u64)
            n235 = Increment(x=w425) -> (x+1=w447:u64)
            n236 = Select(t=w425, s=w440, f=w447) -> (s? t:f=w426:u64)
            n237 = Greater?(x="Number of scans (MCL)", y=w426) -> (0:w433:bool)
            n238 = Multiply(x="Scan freq.  increment (MCL)", y=w443) -> (x*y=w466:i16)
            n239 = Select(t=TRUE, s="Cont. Scan (MCL)", f=w433) -> (s? t:f=w432:bool)
            "Scanning MCL" <- w432
            n240 = Select(t=w426, s=w432, f=w436) -> (s? t:f=w448:u64)
            n241 = feedback-in #20(w448) -> ()
            n242 = Increment(x=w426) -> (x+1=→"Scan I (MCL)":u64)
            n243 = To Word Integer(number=w425) -> (16bit integer=w428:i16)
            n244 = Multiply(x=w428, y="Scan freq.  increment (MCL)") -> (x*y=w427:i16)
          }
        }
        n245 = Select(t=w403, s="1D or 2D Scan?", f=i16 0) -> (s? t:f=w404:i16)
        n246 = Select(t=w404, s="MCL Scan Axis", f=w419) -> (s? t:f=w418:i16)
        n247 = Select(t=w419, s="MCL Scan Axis", f=w404) -> (s? t:f=w420:i16)
        n248 = Add(x=w418, y="AO2") -> (x+y=w407:i16)
        n249 = Add(x="AO1", y=w420) -> (x+y=w408:i16)
        "AO1 2" <- w402
        "AO2 2" <- w401
      }
      frame #3 {
        n250 = feedback-in #21(w489) -> ()
        n251 = feedback #21(w489) -> (w488:u32)
        n252 = Boolean To (0,1)(Boolean="+ phase (MCL)") -> (0, 1=w480:i16)
        n253 = Subtract(x=w489, y=w488) -> (x-y=w487:u32)
        n254 = Multiply(x=w480, y="Phase count adjustment (MCL)") -> (x*y=w476:i16)
        n255 = Subtract(x=w487, y=w486) -> (x-y=w468:u32)
        n256 = Subtract(x="MCL count", y=w468) -> (x-y=w478:u32)
        n257 = feedback #22(i16 0) -> (w477:i16)
        n258 = Subtract(x=w477, y=w476) -> (x-y=w475:i16)
        "MCL Relative Phase" <- w475
        n259 = feedback-in #22(w475) -> ()
        n260 = Number To Boolean Array(number=w468) -> (Boolean array=w469:bool[])
        n261 = Or Array Elements(Boolean array=w469) -> (logical OR=w467:bool)
        "MCL Late?" <- w467
        n262 = Boolean To (0,1)(Boolean=w467) -> (0, 1=w474:i16)
        n263 = Add(x=w478, y=w476) -> (x+y=w482:u32)
        n264 = To Unsigned Word Integer(number=w474) -> (unsigned 16bit integer=w471:u16)
        n265 = feedback #23(u16 0) -> (w472:u16)
        n266 = Add(x=w471, y=w472) -> (x+y=w470:u16)
        "MCL Late Counter" <- w470
        n267 = feedback-in #23(w470) -> ()
      }
    }
    "Numeric" <- w375
  }
  n268 = while "Control APD data integration - stream to host" {
    shift-right: [w493] -> _
    shift-left: w2 -> [w498]
    stop <- FALSE stop-if-true
    n269 = flat-sequence {
      tunnel: w498 -> [w500]
      tunnel: [w501] -> w496
      tunnel: [w500] -> w494
      tunnel: [w509] -> w497
      tunnel: w496 -> [w509]
      tunnel: [w508] -> w495
      tunnel: w494 -> [w508]
      tunnel: [w507] -> w492
      tunnel: [w506] -> w491
      tunnel: [w543] -> w493
      tunnel: w497 -> [w555]
      tunnel: w495 -> [w552]
      tunnel: w492 -> [w536]
      tunnel: w491 -> [w535]
      frame #0 {
        n270 = call "Loop Timer6"("Count(Ticks)"=w500) -> ("Tick Count(Ticks)"=w501:u32)
      }
      frame #1 {
        n271 = flat-sequence {
          tunnel: [w511] -> w505
          tunnel: w505 -> [w513]
          tunnel: [w515] -> w504
          tunnel: [w514] -> w503
          tunnel: [w513] -> w502
          tunnel: [w521] -> w506
          tunnel: [w522] -> w507
          tunnel: w504 -> [w522]
          tunnel: w503 -> [w521]
          tunnel: w502 -> [w520]
          frame #0 {
            # "use two separate variable so each APD won't\nhave to wait to read"
            n272 = feedback #24(FALSE) -> (w510:bool)
            "APD1 out state" <- w510
            "APD2 out state" <- w510
            n273 = Not(x=w510) -> (.not. x?=w511:bool)
            n274 = feedback-in #24(w511) -> ()
          }
          frame #1 {
            n275 = local read "APD 1 Counts 1"() -> (w519:u32)
            n276 = local read "APD 1 Counts 0"() -> (w518:u32)
            n277 = local read "APD 2 Counts 1"() -> (w517:u32)
            n278 = local read "APD 2 Counts 0"() -> (w516:u32)
            n279 = Select(t=w519, s=w513, f=w518) -> (s? t:f=w515:u32)
            n280 = Select(t=w517, s=w513, f=w516) -> (s? t:f=w514:u32)
          }
          frame #2 {
            n281 = case shown="True" w520 {
              frame False {
                w523 = u32 0 ("APD 1 Counts 0")
                n282 = local write "APD 1 Counts 0"(w523) -> ()
                n283 = local write "APD 2 Counts 0"(w523) -> ()
              }
              frame True {
                w524 = u32 0 ("APD 1 Counts 1")
                n284 = local write "APD 1 Counts 1"(w524) -> ()
                n285 = local write "APD 2 Counts 1"(w524) -> ()
              }
            }
          }
        }
      }
      frame #2 {
        n286 = feedback-in #25(w555) -> ()
        n287 = feedback #25(w555) -> (w554:u32)
        n288 = Subtract(x=w555, y=w554) -> (x-y=w553:u32)
        n289 = Subtract(x=w553, y=w552) -> (x-y=w528:u32)
        n290 = case shown="True" "APD to FIFO" {
          tunnel: w536 -> [_ w558]
          tunnel: w535 -> [_ w556]
          frame False {
          }
          frame True {
            n291 = flat-sequence {
              tunnel: 0 ("Timeout") -> [w560]
              tunnel: w558 -> [w561]
              tunnel: [w560] -> w557
              tunnel: w557 -> [w563]
              tunnel: w556 -> [w562]
              frame #0 {
                n292 = xnode ("FIFO Write")("Element"=w561, "Timeout"=w560) -> ()  [unwired: 1 in, 2 out]
              }
              frame #1 {
                n293 = xnode ("FIFO Write")("Element"=w562, "Timeout"=w563) -> ()  [unwired: 1 in, 2 out]
              }
            }
          }
        }
        n294 = Subtract(x="APD Acq Rate Count", y=w528) -> (x-y=w544:u32)
        n295 = Number To Boolean Array(number=w528) -> (Boolean array=w529:bool[])
        n296 = Or Array Elements(Boolean array=w529) -> (logical OR=w527:bool)
        "APD Acq Late?" <- w527
        n297 = Boolean To (0,1)(Boolean=w527) -> (0, 1=w534:i16)
        n298 = To Unsigned Word Integer(number=w534) -> (unsigned 16bit integer=w531:u16)
        n299 = Boolean To (0,1)(Boolean="+ phase (APD Acq)") -> (0, 1=w540:i16)
        n300 = feedback #26(u16 0) -> (w532:u16)
        n301 = Add(x=w531, y=w532) -> (x+y=w530:u16)
        "APD Acq Late Counter" <- w530
        n302 = feedback-in #26(w530) -> ()
        n303 = Multiply(x=w540, y="Phase Count Adjustment (APD Acq)") -> (x*y=w537:i16)
        n304 = Add(x=w544, y=w537) -> (x+y=w543:u32)
        n305 = feedback #27(i16 0) -> (w542:i16)
        n306 = Subtract(x=w542, y=w537) -> (x-y=w539:i16)
        "APD Acq Relative Phase" <- w539
        n307 = feedback-in #27(w539) -> ()
        n308 = To Word Integer(number=w536) -> (16bit integer=w545:i16)
        n309 = To Word Integer(number=w535) -> (16bit integer=w546:i16)
        n310 = Multiply(x="APD 1 AO scale factor", y=w545) -> (x*y=w526:i16)
        n311 = Multiply(x="APD 2 AO scale factor", y=w546) -> (x*y=w525:i16)
        n312 = xnode "FPGA I/O Node"("Connector0/AO6"=w526, "Connector0/AO7"=w525) -> ()  [unwired: 2 in, 2 out]
      }
    }
  }
  n313 = while "Green fluorescent laser interlacing (DO to IA 532 nm AOM ME amp)." {
    shift-right: [w567] -> _
    shift-left: w2 -> [w572]
    shift-right: [w566] -> _
    shift-left: FALSE -> [w564]
    stop <- FALSE stop-if-true
    n314 = flat-sequence {
      tunnel: w572 -> [w575]
      tunnel: [w576] -> w570
      tunnel: [w575] -> w568
      tunnel: [w574] -> w565
      tunnel: w564 -> [w574]
      tunnel: [w579] -> w571
      tunnel: w570 -> [w579]
      tunnel: [w578] -> w569
      tunnel: w568 -> [w578]
      tunnel: w565 -> [w577]
      tunnel: [w588] -> w567
      tunnel: w571 -> [w608]
      tunnel: w569 -> [w605]
      tunnel: [w597] -> w566
      frame #0 {
        n315 = call "Loop Timer4"("Count(Ticks)"=w575) -> ("Tick Count(Ticks)"=w576:u32)
      }
      frame #1 {
        n316 = xnode "FPGA I/O Node"("Connector1/DIO37"=w577, "Connector1/DIO38"=w577, "Connector1/DIO39"=w577) -> ()  [unwired: 3 in, 3 out]
      }
      frame #2 {
        n317 = feedback-in #28(w608) -> ()
        n318 = feedback #28(w608) -> (w607:u32)
        n319 = Subtract(x=w608, y=w607) -> (x-y=w606:u32)
        n320 = Subtract(x=w606, y=w605) -> (x-y=w581:u32)
        n321 = Number To Boolean Array(number=w581) -> (Boolean array=w582:bool[])
        n322 = Or Array Elements(Boolean array=w582) -> (logical OR=w580:bool)
        "GI Late?" <- w580
        n323 = Boolean To (0,1)(Boolean="+ phase (GI)") -> (0, 1=w593:i16)
        n324 = Multiply(x=w593, y="Phase count adjustment (GI)") -> (x*y=w590:i16)
        n325 = Boolean To (0,1)(Boolean=w580) -> (0, 1=w587:i16)
        n326 = To Unsigned Word Integer(number=w587) -> (unsigned 16bit integer=w584:u16)
        n327 = feedback #29(i16 0) -> (w591:i16)
        n328 = feedback #30(u16 0) -> (w585:u16)
        n329 = Add(x=w584, y=w585) -> (x+y=w583:u16)
        "GI Late Counter" <- w583
        n330 = feedback-in #30(w583) -> ()
        n331 = Subtract(x=w591, y=w590) -> (x-y=w589:i16)
        "GI Relative phase" <- w589
        n332 = feedback-in #29(w589) -> ()
        n333 = feedback #31(TRUE) -> (w600:bool)
        n334 = case shown="2" "Operating Mode" {
          tunnel: [TRUE FALSE w614] -> w597
          tunnel: w600 -> [_ _ w611]
          frame 0, Default {
          }
          frame 1 {
          }
          frame 2 {
            n335 = Not(x=w611) -> (.not. x?=w613:bool)
            n336 = Select(t=w613, s="Invert GI", f=w611) -> (s? t:f=w614:bool)
          }
        }
        n337 = Not(x=w600) -> (.not. x?=w596:bool)
        n338 = Select(t="Green interlace ON count", s=w596, f="Green interlace OFF count") -> (s? t:f=w602:u32)
        n339 = Subtract(x=w602, y=w581) -> (x-y=w594:u32)
        n340 = Add(x=w594, y=w590) -> (x+y=w588:u32)
        n341 = feedback-in #31(w596) -> ()
      }
    }
  }
  n342 = while "Green fluorescent laser interlacing (Current to IA 532 nm AOM ME amp)." {
    shift-right: [w620] -> _
    shift-left: w2 -> [w623]
    shift-right: [w617] -> _
    shift-left: u16 0 -> [w615]
    stop <- FALSE stop-if-true
    n343 = flat-sequence {
      tunnel: w623 -> [w626]
      tunnel: [w627] -> w622
      tunnel: [w626] -> w621
      tunnel: [w625] -> w616
      tunnel: w615 -> [w625]
      tunnel: [w630] -> w619
      tunnel: w622 -> [w630]
      tunnel: [w629] -> w618
      tunnel: w621 -> [w629]
      tunnel: w616 -> [w628]
      tunnel: [w639] -> w620
      tunnel: [w656] -> w617
      tunnel: w619 -> [w669]
      tunnel: w618 -> [w666]
      frame #0 {
        n344 = call "Loop Timer10"("Count(Ticks)"=w626) -> ("Tick Count(Ticks)"=w627:u32)
      }
      frame #1 {
        n345 = xnode "FPGA I/O Node"("Chassis2/Mod1/AO0"=w628) -> ()  [unwired: 1 in, 1 out]
      }
      frame #2 {
        n346 = Subtract(x="Green interlace OFF count 2", y="Green int current ON count adj") -> (x-y=w648:u32)
        n347 = feedback-in #32(w669) -> ()
        n348 = feedback #32(w669) -> (w668:u32)
        n349 = Add(x="Green int current ON count adj", y="Green interlace ON count 2") -> (x+y=w649:u32)
        n350 = Subtract(x=w669, y=w668) -> (x-y=w667:u32)
        n351 = Subtract(x=w667, y=w666) -> (x-y=w632:u32)
        n352 = Number To Boolean Array(number=w632) -> (Boolean array=w633:bool[])
        n353 = Boolean To (0,1)(Boolean="+ phase (GI) 2") -> (0, 1=w645:i16)
        n354 = Or Array Elements(Boolean array=w633) -> (logical OR=w631:bool)
        "GI Late? 2" <- w631
        n355 = Boolean To (0,1)(Boolean=w631) -> (0, 1=w638:i16)
        n356 = Multiply(x=w645, y="Phase count adjustment (GI) 2") -> (x*y=w641:i16)
        n357 = To Unsigned Word Integer(number=w638) -> (unsigned 16bit integer=w634:u16)
        n358 = feedback #33(u16 0) -> (w636:u16)
        n359 = Add(x=w634, y=w636) -> (x+y=w635:u16)
        "GI Late Counter 2" <- w635
        n360 = feedback-in #33(w635) -> ()
        n361 = feedback #34(i16 0) -> (w642:i16)
        n362 = Subtract(x=w642, y=w641) -> (x-y=w640:i16)
        "GI Relative phase 2" <- w640
        n363 = feedback-in #34(w640) -> ()
        n364 = feedback #35(TRUE) -> (w661:bool)
        n365 = case shown="0, Default" "Operating Mode 2" {
          tunnel: [TRUE FALSE w686] -> w650
          tunnel: w661 -> [_ _ w683]
          frame 0, Default {
          }
          frame 1 {
          }
          frame 2 {
            n366 = Not(x=w683) -> (.not. x?=w685:bool)
            n367 = Select(t=w685, s="Invert GI 2", f=w683) -> (s? t:f=w686:bool)
          }
        }
        n368 = And(x=w650, y="Green FB On/Off") -> (x .and. y?=w651:bool)
        n369 = case shown="False" w651 {
          tunnel: "Current Out" -> [w670 _]
          tunnel: [w670 w675] -> w655
          frame False {
          }
          frame True {
            n370 = local read "Green FB Sum"() -> (w671:i16)
            n371 = call "Slower PID.vi"("process variable"=w671, "reset?"="Green FB Reset", "setpoint"="Green FB Setpoint", "PID gains (x 2^8)"="Green FB Gains", "output range"=cluster{"output high":i16, "output low":i16} {"output high"=32767, "output low"=-32768} ("Green FB output range")) -> ("output"=w679:i16)  [unwired: 10 out]
            n372 = To Long Integer(number=w679) -> (32bit integer=w672:i32)
            n373 = Add(x=w672, y=32768) -> (x+y=w674:i32)
            n374 = To Unsigned Word Integer(number=w674) -> (unsigned 16bit integer=w675:u16)
          }
        }
        n375 = Not(x=w661) -> (.not. x?=w658:bool)
        n376 = Select(t=w649, s=w658, f=w648) -> (s? t:f=w663:u32)
        n377 = Subtract(x=w663, y=w632) -> (x-y=w643:u32)
        n378 = Add(x=w643, y=w641) -> (x+y=w639:u32)
        n379 = feedback-in #35(w658) -> ()
        n380 = Boolean To (0,1)(Boolean=w650) -> (0, 1=w657:i16)
        n381 = To Unsigned Word Integer(number=w657) -> (unsigned 16bit integer=w654:u16)
        n382 = Multiply(x=w654, y=w655) -> (x*y=w656:u16)
      }
    }
  }
  n383 = while "Green excitation laser feedback measurement" {
    shift-right: [w687] -> _
    shift-left: w2 -> [w692]
    stop <- FALSE stop-if-true
    n384 = flat-sequence {
      tunnel: w692 -> [w694]
      tunnel: [w695] -> w690
      tunnel: [w694] -> w688
      tunnel: [w702] -> w691
      tunnel: w690 -> [w702]
      tunnel: [w701] -> w689
      tunnel: w688 -> [w701]
      tunnel: [w714] -> w687
      tunnel: w691 -> [w725]
      tunnel: w689 -> [w722]
      frame #0 {
        n385 = call "Loop Timer9"("Count(Ticks)"=w694) -> ("Tick Count(Ticks)"=w695:u32)
      }
      frame #1 {
        n386 = xnode "FPGA I/O Node"("Connector1/DIO35"=TRUE) -> ("Chassis2/Mod2/AI0"=w700:i16, "Chassis2/Mod2/AI1"=w699:i16, "Chassis2/Mod2/AI2"=w696:i16)  [unwired: 4 in, 4 out]
        "Green FB Sum" <- w696
        n387 = Bundle("Chassis2/Mod2/AI0"=w700, "Chassis2/Mod2/AI1"=w699, "Chassis2/Mod2/AI2"=w696) -> (→"Green FB Signals":T11)  [unwired: 1 out]
      }
      frame #2 {
        n388 = feedback-in #36(w725) -> ()
        n389 = feedback #36(w725) -> (w724:u32)
        n390 = Subtract(x=w725, y=w724) -> (x-y=w723:u32)
        n391 = xnode "FPGA I/O Node"("Connector1/DIO35"=FALSE) -> ()  [unwired: 1 in, 1 out]
        n392 = Subtract(x=w723, y=w722) -> (x-y=w704:u32)
        n393 = Subtract(x="Green FB Count", y=w704) -> (x-y=w718:u32)
        n394 = Number To Boolean Array(number=w704) -> (Boolean array=w705:bool[])
        n395 = Or Array Elements(Boolean array=w705) -> (logical OR=w703:bool)
        "Green FB Late?" <- w703
        n396 = Boolean To (0,1)(Boolean="+ phase (Green FB)") -> (0, 1=w716:i16)
        n397 = Boolean To (0,1)(Boolean=w703) -> (0, 1=w710:i16)
        n398 = Multiply(x=w716, y="Phase count adjustment (Green FB)") -> (x*y=w711:i16)
        n399 = Add(x=w718, y=w711) -> (x+y=w714:u32)
        n400 = To Unsigned Word Integer(number=w710) -> (unsigned 16bit integer=w707:u16)
        n401 = feedback #37(i16 0) -> (w713:i16)
        n402 = Subtract(x=w713, y=w711) -> (x-y=w712:i16)
        "Green FB Relative Phase" <- w712
        n403 = feedback-in #37(w712) -> ()
        n404 = feedback #38(u16 0) -> (w708:u16)
        n405 = Add(x=w707, y=w708) -> (x+y=w706:u16)
        "Green Late Counter" <- w706
        n406 = feedback-in #38(w706) -> ()
      }
    }
  }
  n407 = while "RF box board DIO control: parallel communication" {
    shift-right: [w732] -> _
    shift-left: w2 -> [w731]
    shift-right: [w730] -> _
    shift-left: FALSE ("Swap F1 and F2") -> [w729]
    stop <- FALSE stop-if-true
    n408 = flat-sequence {
      tunnel: w729 -> [w736]
      tunnel: w731 -> [w734]
      tunnel: [w736] -> w728
      tunnel: [w735] -> w727
      tunnel: [w734] -> w726
      tunnel: [w742] -> w732
      tunnel: [w741] -> w730
      tunnel: w728 -> [w740]
      tunnel: w727 -> [w738]
      tunnel: w726 -> [w737]
      frame #0 {
        n409 = call "Loop Timer"("Count(Ticks)"=w734) -> ("Tick Count(Ticks)"=w735:u32)
      }
      frame #1 {
        n410 = flat-sequence {
          tunnel: ["FPGA Controls\n RF Box"] -> w739
          tunnel: w740 -> [w743]
          tunnel: [w783] -> w742
          tunnel: [w796] -> w741
          tunnel: w739 -> [w795]
          tunnel: w738 -> [w789]
          tunnel: w737 -> [w786]
          frame #0 {
            n411 = case shown="True" "FPGA Controls\n RF Box" {
              tunnel: w743 -> [_ w745]
              frame False {
              }
              frame True {
                n412 = flat-sequence {
                  tunnel: w745 -> [w751]
                  frame #0 {
                    n413 = First Call?() -> (First Call?: T/F=w746:bool)
                    n414 = case shown="True" w746 {
                      frame False {
                      }
                      frame True {
                        # "If first time data updated, be sure to set WR high and UDCLK low\nbefore setting data and address bits."
                        n415 = xnode "FPGA I/O Method Node"("Enable"=TRUE) -> ("FPGA I/O Out"=w748:refnum<k21>)  [unwired: 1 in]
                        n416 = xnode "FPGA I/O Node"("Connector1/DIO15"=TRUE) -> ()  [unwired: 1 in, 1 out]
                        n417 = xnode "FPGA I/O Node"("I/O Item"=FALSE ("Connector1/DIO30"), "FPGA I/O In"=w748) -> ()  [unwired: 1 out]
                      }
                    }
                  }
                  frame #1 {
                    n418 = case shown="True" "Freq or Amp switch first" {
                      tunnel: w751 -> [w753 w758]
                      frame False {
                        n419 = flat-sequence {
                          tunnel: w753 -> [w757]
                          frame #0 {
                            # "switch amplitude"
                            # "send udclk high"
                            n420 = xnode "FPGA I/O Node"("Connector1/DIO30"=TRUE ("Connector1/DIO15")) -> ()  [unwired: 1 in, 1 out]
                          }
                          frame #1 {
                            # "send udclk low"
                            n421 = xnode "FPGA I/O Node"("Connector1/DIO30"=FALSE ("Connector1/DIO15")) -> ()  [unwired: 1 in, 1 out]
                          }
                          frame #2 {
                            n422 = call "Wait5"("Count(Ticks)"="Freq switch delay") -> ()  [unwired: 1 out]
                          }
                          frame #3 {
                            # "switch frequency"
                            n423 = xnode "FPGA I/O Node"("Connector1/DIO36"=w757) -> ()  [unwired: 1 in, 1 out]
                          }
                        }
                      }
                      frame True {
                        n424 = flat-sequence {
                          tunnel: w758 -> [w759]
                          frame #0 {
                            # "switch frequency"
                            n425 = xnode "FPGA I/O Node"("Connector1/DIO36"=w759) -> ()  [unwired: 1 in, 1 out]
                          }
                          frame #1 {
                            n426 = call "Wait4"("Count(Ticks)"="Amp switch delay") -> ()  [unwired: 1 out]
                          }
                          frame #2 {
                            # "switch amplitude"
                            # "send udclk high"
                            n427 = xnode "FPGA I/O Node"("Connector1/DIO30"=TRUE ("Connector1/DIO15")) -> ()  [unwired: 1 in, 1 out]
                          }
                          frame #3 {
                            # "send udclk low"
                            n428 = xnode "FPGA I/O Node"("Connector1/DIO30"=FALSE ("Connector1/DIO15")) -> ()  [unwired: 1 in, 1 out]
                          }
                        }
                      }
                    }
                  }
                }
              }
            }
          }
          frame #1 {
            # "This is the prior cycle's on time"
            # "increment timing\nindex, reset to 0 if \nend of matrix"
            # "Reset to begginning (1) when number of cycles reached."
            # "timing index"
            # "build byte stacks for writing data\n(must correspond to addresses array constant)"
            # "Timing housekeeping"
            # "Adjust phase if late\n(maintains constant phase relationship between cycles)"
            n429 = feedback #39(u8 0 ("t")) -> (w792:u8)
            n430 = Increment(x=w792) -> (x+1=w836:u8)
            n431 = Increment(x="Number Interlace Cycles") -> (x+1=w831:u8)
            n432 = Equal?(x=w836, y=w831) -> (x = y?=w838:bool)
            n433 = Select(t=u8 1, s=w838, f=w836) -> (s? t:f=w791:u8)
            n434 = feedback-in #39(w791) -> ()
            n435 = Increment(x=w791) -> (x+1=w833:u8)
            n436 = Equal?(x=w833, y=w831) -> (x = y?=w834:bool)
            n437 = Select(t=u8 1, s=w834, f=w833) -> (s? t:f=w830:u8)
            n438 = Select(t=w830, s="Interlace ON/OFF", f="Interlace Off Parameters") -> (s? t:f=w814:u8)
            n439 = case shown="1, Default" w814 {
              tunnel: [w887 "BD 1 Frequency 2" "BD 1 Frequency 3"] -> w826
              tunnel: [w886 "BD 2 Frequency 2" "BD 2 Frequency 3"] -> w815
              tunnel: ["BD 2 Amplitude 1" "BD 2 Amplitude 2" "BD 2 Amplitude 3"] -> w771
              tunnel: [w875 w1012 "BD 1 Amplitude 3"] -> w774
              frame 1, Default {
                w882 = u64 0 ("f")
                # "Trap 1"
                n440 = local read "Scanning"() -> (w888:bool)
                n441 = case "For position feedback" shown="True" "Force feedback" {
                  tunnel: [i64 0 w906] -> w872
                  frame False {
                  }
                  frame True {
                    w897 = fxp<+/-,24,9> 0.0 ("AI1 X Set 2")
                    w909 = u16 0
                    n442 = local read "AI1 X Set 2"() -> (w903:fxp<+/-,16,1>)
                    n443 = local read "AI1 X Set 1"() -> (w902:fxp<+/-,16,1>)
                    n444 = feedback #40(w909) -> (w910:u16)
                    n445 = Increment(x=w910) -> (x+1=w908:u16)
                    n446 = Select(t=w902, s="Trap Pos FB Monitor T1 or T2", f=w903) -> (s? t:f=w899:fxp<+/-,16,1>)
                    n447 = Greater Or Equal?(x=w908, y="Trap Pos FB Int Count") -> (x >= y?=w900:bool)
                    n448 = Select(t=w909, s=w900, f=w908) -> (s? t:f=w907:u16)
                    n449 = feedback-in #40(w907) -> ()
                    n450 = feedback #41(w897) -> (w898:fxp<+/-,24,9>)
                    n451 = Add(x=w899, y=w898) -> (x+y=w894:fxp<+/-,24,9>)
                    n452 = Select(t=w897, s=w900, f=w894) -> (s? t:f=w896:fxp<+/-,24,9>)
                    n453 = feedback-in #41(w896) -> ()
                    n454 = feedback #42(i64 0) -> (w905:i64)
                    n455 = case shown="True" w900 {
                      tunnel: [w911 w925] -> w906
                      tunnel: w905 -> [w911 _]
                      tunnel: "Trap Pos FB Int Count" -> [_ w913]
                      tunnel: w894 -> [_ w914]
                      frame False {
                      }
                      frame True {
                        n456 = Divide(x=w914, y=w913) -> (x/y=w912:fxp<+/-,16,1>)
                        "Trap Pos FB Int-Norm Signal" <- w912
                        n457 = xnode ("PID")("process variable"=w912, "reset?"="Trap Pos. FB Reset", "setpoint"="Trap Pos. FB SP", "PID gains"="Trap Pos. FB Gains", "output range"="Trap Pos. FB Range") -> ("output"=w923:fxp<+/-,16,1>)
                        n458 = Negate(x=w923) -> (-x=w922:fxp<+/-,17,2>)
                        n459 = Select(t=w922, s="Trap Pos FB Negate Action", f=w923) -> (s? t:f=w919:fxp<+/-,17,2>)
                        n460 = Scale By Power Of 2(n=u32 15, x=u32 1) -> (x*2^n=w916:u32)
                        n461 = Multiply(x=w919, y=w916) -> (x*y=w915:fxp<+/-,17,17>)
                        n462 = To Quad Integer(1:w915) -> (0:w928:i64)
                        "Trap Pos FB Action" <- w928
                        n463 = Multiply(x=w928, y="Trap Pos. FB Mult Factor") -> (x*y=w926:i64)
                        n464 = Add(x=w926, y="Trap Pos. FB Offset Factor") -> (x+y=w925:i64)
                        "Trap Pos FB Int Signal" <- w914
                      }
                    }
                    n465 = feedback-in #42(w906) -> ()
                  }
                }
                n466 = Or(x=w888, y="Start scan") -> (x .or. y?=w880:bool)
                n467 = Not(x="Abort scan") -> (.not. x?=w878:bool)
                n468 = And(x=w878, y=w880) -> (x .and. y?=w877:bool)
                n469 = case "For raster scanning" shown="False" w877 {
                  tunnel: [u64 0 w1000] -> w883
                  tunnel: "Start scan" -> [_ w985]
                  frame False {
                    n470 = local write "Scanning"(FALSE ("scanning")) -> ()
                  }
                  frame True {
                    w969 = i64 0
                    w968 = u64 0
                    # "scan incr."
                    # "freq. incr. mult."
                    # "count steps"
                    # "count number of cycles"
                    n471 = feedback #43(w968) -> (w997:u64)
                    n472 = Select(t=w968, s=w985, f=w997) -> (s? t:f=w999:u64)
                    n473 = Increment(x=w999) -> (x+1=w996:u64)
                    n474 = Greater?(x="Cycles per step", y=w996) -> (0:w978:bool)
                    n475 = Select(t=w996, s=w978, f=w968) -> (s? t:f=w995:u64)
                    n476 = feedback-in #43(w995) -> ()
                    n477 = feedback #44(w968) -> (w994:u64)
                    n478 = Select(t=w968, s=w985, f=w994) -> (s? t:f=w989:u64)
                    n479 = Increment(x=w989) -> (x+1=w993:u64)
                    n480 = Add(x="Scan steps", y="Scan steps") -> (x+y=w992:u64)
                    n481 = Select(t=w989, s=w978, f=w993) -> (s? t:f=w973:u64)
                    n482 = Greater?(x=w992, y=w973) -> (0:w972:bool)
                    n483 = Select(t=w973, s=w972, f=w968) -> (s? t:f=w990:u64)
                    n484 = feedback-in #44(w990) -> ()
                    n485 = Equal?(x="Scan steps", y=w973) -> (x = y?=w977:bool)
                    n486 = Greater?(x="Scan steps", y=w989) -> (0:w988:bool)
                    n487 = feedback #45(w969) -> (w991:i64)
                    n488 = Select(t=w969, s=w985, f=w991) -> (s? t:f=w975:i64)
                    n489 = Increment(x=w975) -> (x+1=w987:i64)
                    n490 = Decrement(x=w975) -> (x-1=w986:i64)
                    n491 = Select(t=w987, s=w988, f=w986) -> (s? t:f=w976:i64)
                    n492 = Select(t=w975, s=w977, f=w976) -> (s? t:f=w974:i64)
                    n493 = Select(t=w975, s=w978, f=w974) -> (s? t:f=w970:i64)
                    n494 = Select(t=w970, s=w972, f=w969) -> (s? t:f=w971:i64)
                    n495 = feedback-in #45(w971) -> ()
                    n496 = feedback #46(w968) -> (w984:u64)
                    n497 = Select(t=w968, s=w985, f=w984) -> (s? t:f=w980:u64)
                    n498 = Increment(x=w980) -> (x+1=w981:u64)
                    n499 = Select(t=w980, s=w972, f=w981) -> (s? t:f=w979:u64)
                    n500 = Greater?(x="Number of scans", y=w979) -> (0:w965:bool)
                    n501 = Multiply(x="Scan freq.  increment", y=w975) -> (x*y=w1000:i64)
                    n502 = Select(t=TRUE, s="Cont. Scan", f=w965) -> (s? t:f=w964:bool)
                    "Scanning" <- w964
                    n503 = Select(t=w979, s=w964, f=w968) -> (s? t:f=w982:u64)
                    n504 = feedback-in #46(w982) -> ()
                    n505 = Increment(x=w979) -> (x+1=→"Scan I":u64)
                  }
                }
                n506 = case "For intensity feedback" shown="True" "FB On/Off Set 1" {
                  tunnel: "BD 1 Amplitude 1" -> [w1002 _]
                  tunnel: [w1002 w1003] -> w875
                  frame False {
                  }
                  frame True {
                    n507 = local read "AI2 Y Sum Set 1"() -> (w1005:i16)
                    n508 = call "Slower PID.vi"("process variable"=w1005, "reset?"="FB Reset Set 1", "setpoint"="FB Setpoint Set 1", "PID gains (x 2^8)"="FB Gains Set 1", "output range"="FB output range 1") -> ("output"=w1008:i16)  [unwired: 10 out]
                    n509 = To Unsigned Word Integer(number=w1008) -> (unsigned 16bit integer=w1003:u16)
                  }
                }
                n510 = Select(t=w882, s="Scan BD", f=w883) -> (s? t:f=w881:u64)
                n511 = Select(t=w883, s="Scan BD", f=w882) -> (s? t:f=w884:u64)
                n512 = Add(x=w881, y="BD 2 Frequency 1") -> (x+y=w886:u64)
                n513 = Compound Arithmetic op=ADD("BD 1 Frequency 1", w872, w884) -> (w887:u64)
                "BD1 Frequency Out 1" <- w887
              }
              frame 2 {
                # "Trap 2"
                n514 = case shown="True" "FB On/Off Set 2" {
                  tunnel: [w1016 w1017] -> w1012
                  tunnel: "BD 1 Amplitude 2" -> [w1016 _]
                  frame False {
                  }
                  frame True {
                    n515 = local read "AI2 Y Sum Set 2"() -> (w1022:i16)
                    n516 = call "Slower PID.vi"("process variable"=w1022, "reset?"="FB Reset Set 2", "setpoint"="FB Setpoint Set 2", "PID gains (x 2^8)"="FB Gains Set 2", "output range"="FB output range 2") -> ("output"=w1019:i16)  [unwired: 10 out]
                    n517 = To Unsigned Word Integer(number=w1019) -> (unsigned 16bit integer=w1017:u16)
                  }
                }
                "BD1 Frequency Out 2" <- "BD 1 Frequency 2"
              }
              frame 3 {
                # "Fluorescence period"
              }
            }
            n518 = feedback-in #47(w789) -> ()
            n519 = feedback #47(w789) -> (w788:u32)
            n520 = Select(t=w791, s="Interlace ON/OFF", f="Interlace Off Parameters") -> (s? t:f=w829:u8)
            n521 = Subtract(x=w789, y=w788) -> (x-y=w787:u32)
            n522 = Subtract "The error"(x=w787, y=w786) -> (x-y=w764:u32)
            n523 = case shown="1, Default" w829 {
              tunnel: ["DIO count 1 (ticks)" "DIO count 2 (ticks)" "DIO count 3 (ticks)"] -> w785
              frame 1, Default {
              }
              frame 2 {
              }
              frame 3 {
              }
            }
            n524 = Number To Boolean Array(number=w764) -> (Boolean array=w765:bool[])
            n525 = Or Array Elements(Boolean array=w765) -> (logical OR=w763:bool)
            "DIO Late?" <- w763
            n526 = Boolean To (0,1)(Boolean=w763) -> (0, 1=w770:i16)
            n527 = To Unsigned Word Integer(number=w770) -> (unsigned 16bit integer=w767:u16)
            n528 = feedback #48(u16 0) -> (w768:u16)
            n529 = Add(x=w767, y=w768) -> (x+y=w766:u16)
            "DIO Late Counter" <- w766
            n530 = feedback-in #48(w766) -> ()
            n531 = Subtract(x=w785, y=w764) -> (x-y=w784:u32)
            n532 = Split Number(x=w826) -> (hi(x)=w825:u32, lo(x)=w824:u32)
            n533 = Split Number(x=w815) -> (hi(x)=w820:u32, lo(x)=w819:u32)
            n534 = Boolean To (0,1)(Boolean="+ phase (DIO)") -> (0, 1=w781:i16)
            n535 = Split Number(x=w825) -> (lo(x)=w823:u16)  [unwired: 1 out]
            n536 = Split Number(x=w824) -> (hi(x)=w822:u16, lo(x)=w821:u16)
            n537 = Split Number(x=w820) -> (lo(x)=w818:u16)  [unwired: 1 out]
            n538 = Split Number(x=w819) -> (hi(x)=w817:u16, lo(x)=w816:u16)
            n539 = Split Number(x=w774) -> (hi(x)=w776:u8, lo(x)=w775:u8)
            n540 = Split Number(x=w771) -> (hi(x)=w773:u8, lo(x)=w772:u8)
            n541 = Split Number(x=w823) -> (hi(x)=w813:u8, lo(x)=w812:u8)
            n542 = Split Number(x=w822) -> (hi(x)=w811:u8, lo(x)=w810:u8)
            n543 = Split Number(x=w818) -> (hi(x)=w806:u8, lo(x)=w805:u8)
            n544 = Split Number(x=w821) -> (hi(x)=w809:u8, lo(x)=w808:u8)
            n545 = Split Number(x=w817) -> (hi(x)=w804:u8, lo(x)=w803:u8)
            n546 = Split Number(x=w816) -> (hi(x)=w802:u8, lo(x)=w801:u8)
            n547 = Multiply(x=w781, y="Phase count adjustment (DIO)") -> (x*y=w777:i16)
            n548 = feedback #49(i16 0) -> (w779:i16)
            n549 = Subtract(x=w779, y=w777) -> (x-y=w778:i16)
            "DIO Relative phase" <- w778
            n550 = feedback-in #49(w778) -> ()
            n551 = Add(x=w784, y=w777) -> (x+y=w783:u32)
            n552 = Build Array "BD 1 A Stack"(w776, w775) -> (w798:u8[])
            n553 = Build Array "BD 2 A Stack"(w773, w772) -> (w797:u8[])
            n554 = Build Array "BD 1 nu Stack"(w813, w812, w811, w810, w809, w808) -> (w807:u8[])
            n555 = Build Array "BD 2 nu Stack"(w806, w805, w804, w803, w802, w801) -> (w800:u8[])
            n556 = case shown="1, Default" w814 {
              tunnel: [w864 w867] -> w796
              tunnel: [u8 10 u8 4] -> w799
              tunnel: "Swap F1 and F2" -> [w865 w867]
              frame 2 {
                # "F2"
                n557 = Not(x=w865) -> (.not. x?=w864:bool)
              }
              frame 1, Default {
                # "low chooses F1"
                # "F1"
              }
            }
            n558 = case "If FPGA is controlling (toggling) RF synth" shown="True" w795 {
              tunnel: w807 -> [_ w843]
              tunnel: w800 -> [_ w842]
              tunnel: w799 -> [_ w841]
              tunnel: w798 -> [_ w840]
              tunnel: w797 -> [_ w839]
              frame False {
              }
              frame True {
                # "Write next amp.\n(wait until beginning of next loop iteration to update)"
                n559 = flat-sequence "Update the next F1 and F2 frequency value (the actual frequency won't change until FSK is switched).\nThen load the next amplitude value into buffer, but don't update it until the next cycle." {
                  tunnel: w843 -> [w846]
                  tunnel: w842 -> [w845]
                  tunnel: w841 -> [w844]
                  tunnel: w840 -> [w857]
                  tunnel: w839 -> [w856]
                  frame #0 {
                    n560 = for {
                      tunnel: w846 -> [w852] mode=indexing
                      tunnel: w845 -> [w851] mode=indexing
                      tunnel: w844 -> [w849]
                      i -> [w850]
                      # "Write next freq."
                      n561 = To Unsigned Byte Integer(number=w850) -> (unsigned 8bit integer=w847:u8)
                      n562 = Add(x=w849, y=w847) -> (x+y=w848:u8)
                      n563 = call "write to RF synth bd.vi"("Address Byte"=w848, "BD 2 Byte"=w851, "BD 1 Byte"=w852) -> ()  [unwired: 2 in]
                    }
                  }
                  frame #1 {
                    # "send udclk high"
                    n564 = xnode "FPGA I/O Node"("Connector1/DIO30"=TRUE ("Connector1/DIO15")) -> ()  [unwired: 1 in, 1 out]
                  }
                  frame #2 {
                    n565 = xnode "FPGA I/O Node"("Connector1/DIO30"=FALSE ("Connector1/DIO15")) -> ()  [unwired: 1 in, 1 out]
                  }
                  frame #3 {
                    n566 = for {
                      tunnel: w857 -> [w863] mode=indexing
                      tunnel: w856 -> [w862] mode=indexing
                      tunnel: u8 33 -> [w860]
                      i -> [w861]
                      n567 = To Unsigned Byte Integer(number=w861) -> (unsigned 8bit integer=w858:u8)
                      n568 = Add(x=w860, y=w858) -> (x+y=w859:u8)
                      n569 = call "write to RF synth bd.vi"("Address Byte"=w859, "BD 2 Byte"=w862, "BD 1 Byte"=w863) -> ()  [unwired: 2 in]
                    }
                  }
                }
              }
            }
          }
        }
      }
    }
  }
  n570 = node-c288(w4) -> ()
